vi "test_LockIn.vi"() -> ()   [LabVIEW 2014]
uses:
  <instrlib>/Zurich Instruments LabOne/Public/Data/ziTypePollType.ctl
  <instrlib>/Zurich Instruments LabOne/Zurich Instruments LabOne.lvlib
panel:
  out "ziValueType":T1
  out "Value Int":i32
  out "Value Double":dbl
  out "PathArray":string[](array[string])
  out "error out":errorcluster
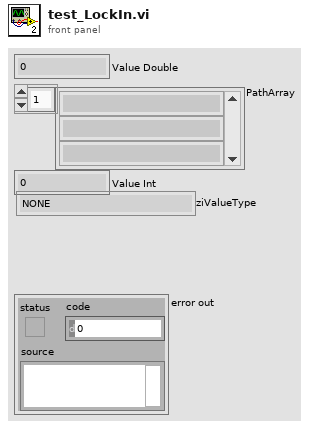
[diagram p1: front panel]
types:
  T1 = typedef "Zurich Instruments LabOne.lvlib/ziTypePollType.ctl" = enum16{"NONE", "DOUBLE_DATA", "INTEGER_DATA", "DEMOD_SAMPLE", "SCOPE_WAVE_HF2", "AUXIN_SAMPLE", "DIO_SAMPLE", "BYTE_ARRAY", "PWA_WAVE", "9", "10", "11", "12", "13", "14", "15", "TREE_CHANGE_DEPRI", "17", "ERROR", "19", "20", "21", "22", "23", "24", "25", "26", "27", "28", "29", "30", "31", "DOUBLE_DATA_TS", "INTEGER_DATA_TS", "34", "SCOPE_WAVE", "36", "37", "BYTE_ARRAY_TS", "39", "40", "41", "42", "43", "44", "45", "46", "47", "TREE_CHANGE"}
  T2 = typedef "Zurich Instruments LabOne.lvlib/ziTypeHandle.ctl" = cluster{"handleValid":bool, "Conn":u64, "Path Prefix":string, "EventBuffer":u8[], "Connected":bool, "Clockbase(s)":dbl}
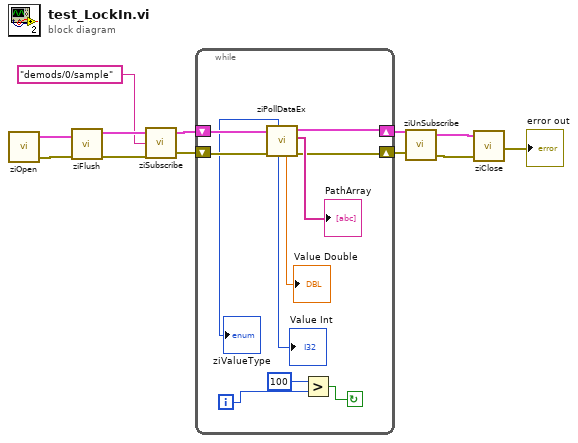
[diagram p0: block diagram]
diagram:
  n1 = call <instrlib>:"ziOpen.vi"() -> ("Error Out"=w11:errorcluster, "HandleOut"=w12:T2)  [unwired: 4 in, 1 out]
  n2 = call <instrlib>:"ziFlush.vi"("error in"=w11, "Handle In"=w12) -> ("error out"=w10:errorcluster, "Handle Out"=w9:T2)  [unwired: 8 in]
  n3 = call <instrlib>:"ziSubscribe.vi"("error in"=w10, "Path ()"="demods/0/sample", "Handle In"=w9) -> ("error out"=w7:errorcluster, "Handle Out"=w8:T2)  [unwired: 1 in]
  n4 = while {
    shift-right: [w17] -> w6
    shift-left: w8 -> [w20]
    shift-right: [w16] -> w5
    shift-left: w7 -> [w19]
    i -> [w23]
    stop <- w22 continue-if-true
    n5 = call <instrlib>:"ziPollDataEx.vi"("error in"=w19, "Handle In"=w20) -> ("error out"=w16:errorcluster, "PathArray"=→"PathArray":string[], "Handle Out"=w17:T2, "Value Double"=→"Value Double":dbl, "Value Int"=→"Value Int":i32, "ziValueType"=→"ziValueType":T1)  [unwired: 2 in, 2 out]
    n6 = Greater?(x=100, y=w23) -> (0:w22:bool)
  }
  n7 = call <instrlib>:"ziUnSubscribe.vi"("error in"=w5, "Handle in"=w6) -> ("error out"=w2:errorcluster, "Handle out"=w3:T2)  [unwired: 2 in]
  n8 = call <instrlib>:"ziClose.vi"("Error In"=w2, "Handle In"=w3) -> ("Error Out"=→"error out":errorcluster)  [unwired: 2 in, 1 out]
